vi "3D Stem Graph.vi"() -> ()   [LabVIEW 2023]
doc: "This VI shows how to use the 3D Stem Plot."
uses:
  <vilib>/Math Plots/3D Math Plots/3D Stem/3D Stem XCtrl/3D Stem.xctl
  <vilib>/Math Plots/3D Math Plots/3D Stem/3D Stem Datatype/Public/Plot Helper (Vector).vi
  <vilib>/Math Plots/3D Math Plots/3D Stem/3D Stem Datatype/3D Stem Datatype.lvclass
panel:
  out "3D Stem":refnum<class "3D Plot Datatype.lvclass">[](xcontrol)
  # "Overview: Demonstrates the Stem indicator from the Graph > 3D Graph palette.\nRequirements: LabVIEW Full Development System\nInstructions:\nRun the VI."
  # "Try the following operations on the graph:\n\n1. Click and drag the mouse within the graph to change the view direction.\n2. Press the Shift key and drag the mouse up to zoom in.\n3. Press the Shift key and drag the mouse down to zoom out.\n4. Right-click the graph and choose 3D Plot Properties to configure various properties related to the graph's appearance.\n5. Right-click the graph and select Export Image >Export to File."
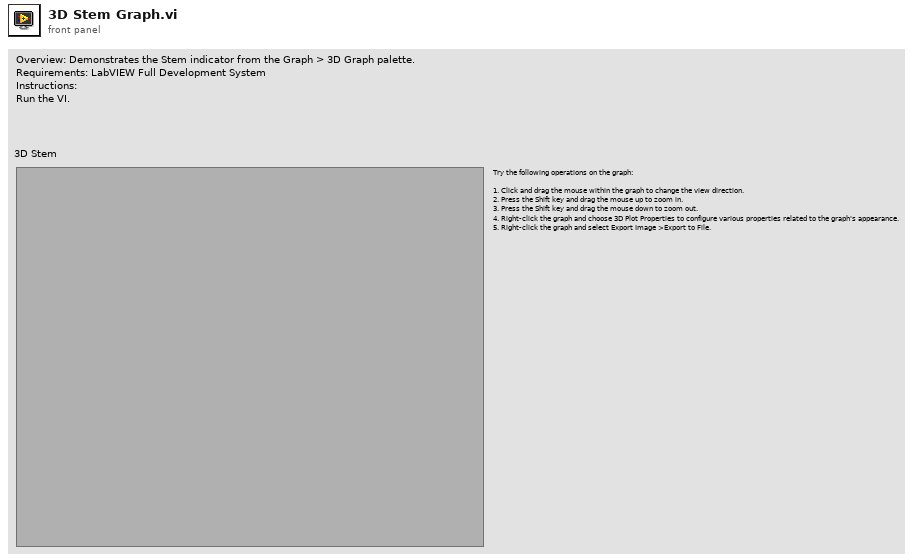
[diagram p1: front panel]
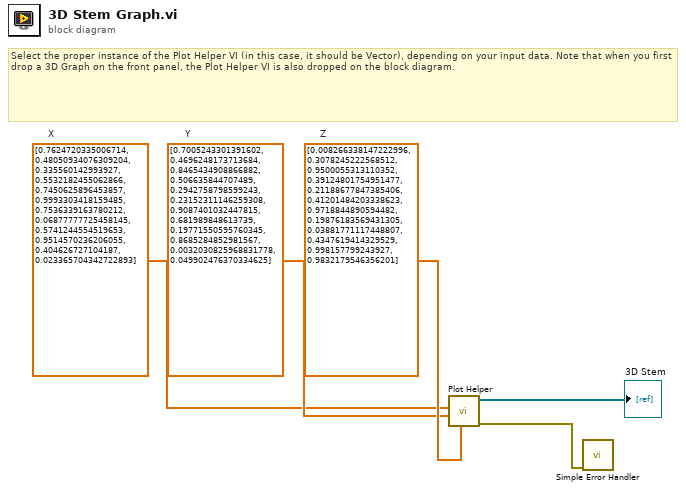
[diagram p0: block diagram]
diagram:
  w5 = sgl[] [0.008266338, 0.30782452, 0.95000553, 0.39124802, 0.21188678, 0.41201484, 0.9718845, 0.19876184, 0.03881771, 0.43476194, 0.9981578, 0.98321795]  # Z
  w4 = sgl[] [0.70052433, 0.46962482, 0.8465435, 0.50663584, 0.29427588, 0.23152311, 0.9087401, 0.68198985, 0.1977155, 0.8685285, 0.0032030826, 0.049902476]  # Y
  w3 = sgl[] [0.76247203, 0.48050934, 0.33556014, 0.55321825, 0.7450626, 0.99933034, 0.7536339, 0.06877778, 0.57412446, 0.951457, 0.40462673, 0.023365704]  # X
  # "Select the proper instance of the Plot Helper VI (in this case, it should be Vector), depending on your input data. Note that when you first drop a 3D Graph on the front panel, the Plot Helper VI is also dropped on the block diagram."
  n1 = call-poly <vilib>:"Plot Helper.vi"("z vector"=w5, "y vector"=w4, "x vector"=w3) -> ("error out"=w1:errorcluster, "3D Plot lvclass Array out"=→"3D Stem":refnum<class "3D Plot Datatype.lvclass">[])  [unwired: 3 in, 4 out]
  n2 = call <vilib>:"Simple Error Handler.vi"("error in (no error)"=w1) -> ()  [unwired: 4 in, 5 out]
